vi "tearDown.vi"(8 "error in (no error)":errorcluster, 11 "reference in":refnum<class "Embedded Data Logger Scripting Unit Tests.lvclass">) -> (0 "error out":errorcluster, 3 "reference out":refnum<class "Embedded Data Logger Scripting Unit Tests.lvclass">)   [LabVIEW 2027, in "Embedded Data Logger Scripting Unit Tests.lvclass"]
doc: "tearDown runs after the test method has completed. Use this method to clean up any operations or references that were opened by setUp or the test method. Unit tests should be independent of other unit tests so this VI should ensure that the next test can run in a 'clean' test environment."
uses:
  Embedded Data Logger Scripting Unit Tests.lvclass
  C:/Program Files/National Instruments/LabVIEW 2027/vi.lib/NI/VeriStand Custom Device Testing Tools/VeriStandScriptingTestCase/VeriStandScriptingTestCase.lvclass
  <vilib>/NI/VeriStand Custom Device Testing Tools/VeriStandScriptingTestCase/VeriStandScriptingTestCase.lvclass
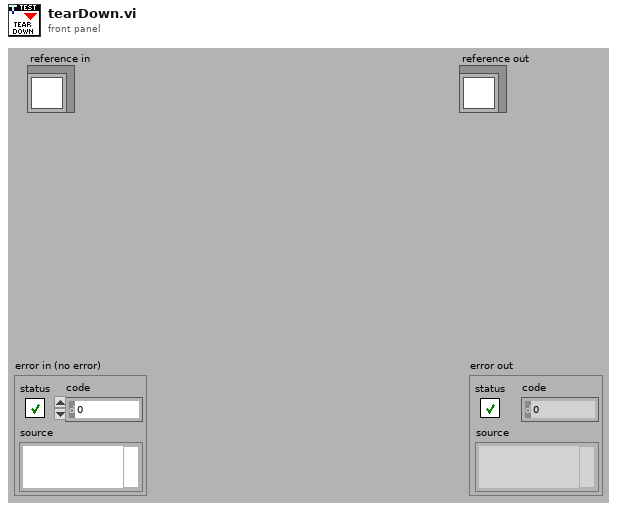
[diagram p1: front panel]
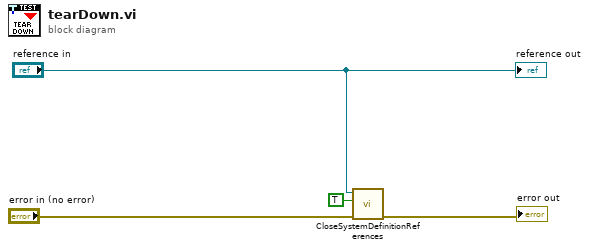
[diagram p0: block diagram]
diagram:
  n1 = call <vilib>:"CloseSystemDefinitionReferences.vi"("error in"="error in (no error)", "Delete Sysdef? (F)"=TRUE, "VeriStandScriptingTestCase in"="reference in") -> ("error out"=→"error out":errorcluster)  [unwired: 7 in, 1 out]
  "reference out" <- "reference in"
